vi "Write Resource.vi"(8 "error in (no error)":errorcluster, 10 "Resource":variant, 11 "Generic Controller in":refnum<class "Generic Plugin.lvclass">) -> (0 "error out":errorcluster, 3 "Generic Controller out":refnum<class "Generic Plugin.lvclass">)   [LabVIEW 2020, in "Generic Plugin.lvclass"]
uses:
  Generic Plugin.lvclass
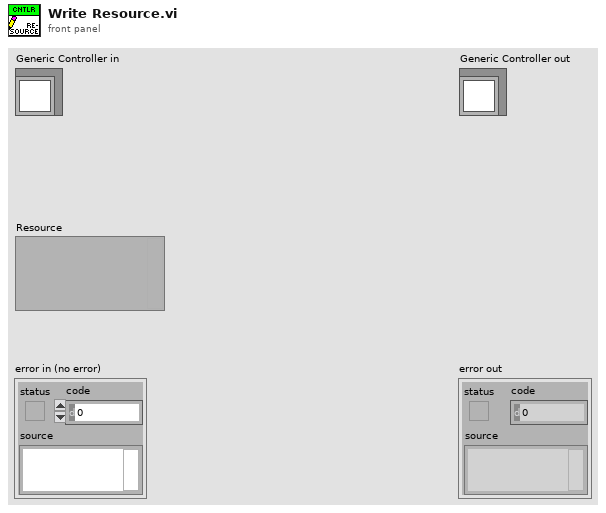
[diagram p1: front panel]
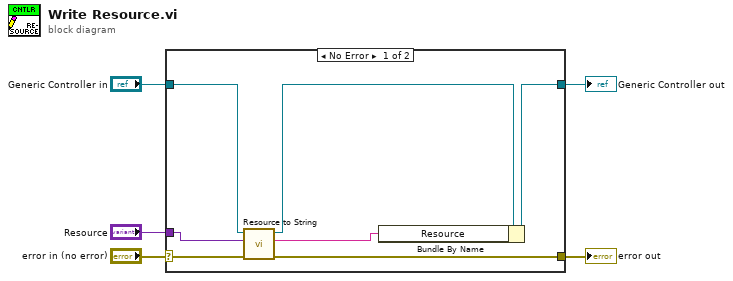
[diagram p0: block diagram]
diagram:
  n1 = case shown="No Error" "error in (no error)" {
    selector: "error in (no error)" -> [w11 w13]
    tunnel: [w10 w13] -> w4
    tunnel: [w12 w14] -> w2
    tunnel: "Generic Controller in" -> [w7 w14]
    tunnel: "Resource" -> [w9 _]
    frame No Error {
      n2 = call-dynamic "Resource to String.vi"("error in (no error)"=w11, "Resource as Variant"=w9, "Generic Controller in"=w7) -> ("error out"=w10:errorcluster, "Resource as String"=w8:string, "Generic Controller out"=w6:refnum<class "Generic Plugin.lvclass">)  [unwired: 6 in]
      n3 = Bundle By Name(cluster=w6, "Resource"=w8) -> (w12:refnum<class "Generic Plugin.lvclass">)
    }
    frame Error {
    }
  }
  "error out" <- w4
  "Generic Controller out" <- w2
